vi "Send ABORT.vi"(8 "error in (no error)":errorcluster, 9 "Abort Request":T1, 11 "WAMP Client in":refnum<class "WAMP Client.lvclass">) -> (0 "error out":errorcluster, 3 "WAMP Client out":refnum<class "WAMP Client.lvclass">)   [LabVIEW 2020, in "wamplv.lvlib" / "WAMP Client.lvclass"]
uses:
  WAMP Client.lvclass
  API/TypeDefs/Termination Reason.ctl
  TypeDef/Termination Reason Enum.ctl
  WAMP Client.lvclass/WAMP Client.ctl
  Private/Comm Handlers/ICommHandler/ICommHandler.lvclass
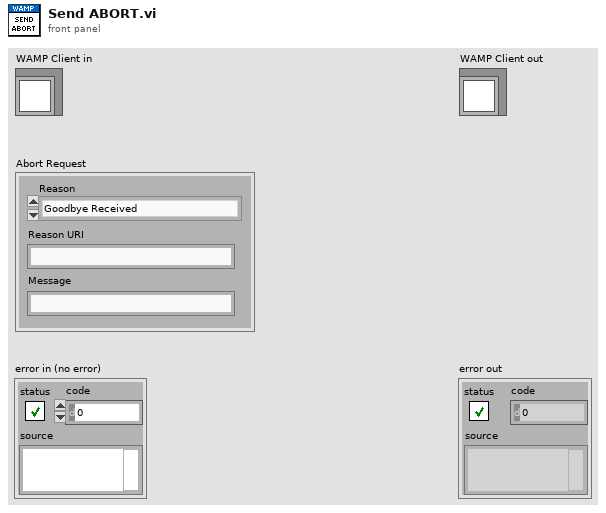
[diagram p1: front panel]
types:
  T1 = typedef "wamplv.lvlib/WAMP Client.lvclass/Termination Reason.ctl" = cluster{"Reason":T2, "Reason URI":string, "Message":string}
  T2 = typedef "wamplv.lvlib/WAMP Client.lvclass/Termination Reason Enum.ctl" = enum16{"Goodbye Received", "Abort Received", "Send Goodbye", "Send Abort", "Read Loop Failure", "Write Loop Failure", "Message Loop Failure"}
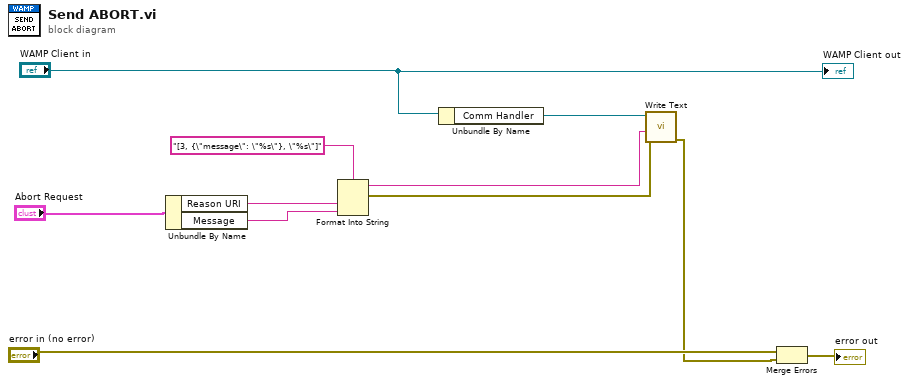
[diagram p0: block diagram]
diagram:
  n1 = Unbundle By Name("Abort Request") -> ("Reason URI"=w8:string, "Message"=w7:string)
  n2 = Format Into String(format string="[3, {\"message\": \"%s\"}, \"%s\"]", w8, w7) -> (resulting string=w5:string, error out=w4:errorcluster)  [unwired: 2 in]
  n3 = Unbundle By Name("WAMP Client in") -> ("Comm Handler"=w9:refnum<class "ICommHandler.lvclass">)
  n4 = call-dynamic "Write Text.vi"("error in (no error)"=w4, "String"=w5, "ICommHandler in"=w9) -> ("error out"=w1:errorcluster)  [unwired: 7 in, 1 out]
  n5 = Merge Errors("error in (no error)", w1) -> (→"error out":errorcluster)
  "WAMP Client out" <- "WAMP Client in"
